vi "Timing.vi"(5 "Tag Values":string[](array[string]), 7 "Tags":string[](array[string]), 8 "error in (no error)":errorcluster, 9 "Time (ms)":u32, 10 "Metric Name":string, 11 "StatD Interface in":refnum<class "StatD Interface.lvclass">) -> (0 "error out":errorcluster, 3 "StatD Interface out":refnum<class "StatD Interface.lvclass">)   [LabVIEW 2011, in "StatD Interface.lvclass"]
doc: "Record a time measurement."
uses:
  StatD Interface.lvclass
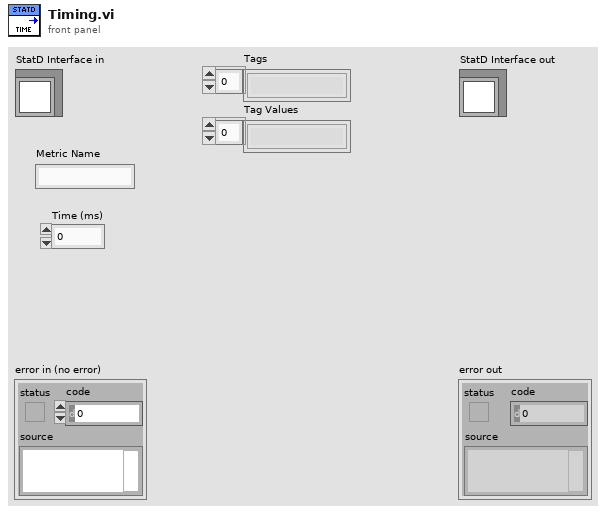
[diagram p1: front panel]
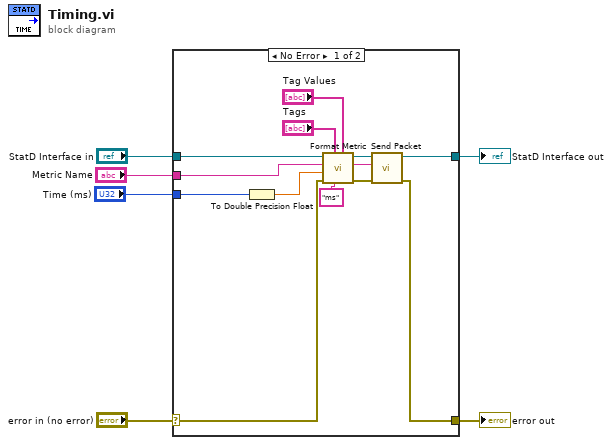
[diagram p0: block diagram]
diagram:
  n1 = case shown="No Error" "error in (no error)" {
    selector: "error in (no error)" -> [w8 w21]
    tunnel: [w18 w21] -> w5
    tunnel: [w19 w20] -> w3
    tunnel: "StatD Interface in" -> [w14 w20]
    tunnel: "Time (ms)" -> [w10 _]
    tunnel: "Metric Name" -> [w9 _]
    frame No Error {
      n2 = To Double Precision Float(number=w10) -> (double precision float=w7:dbl)
      n3 = call "Format Metric.vi"("Tag Values"="Tag Values", "Metric Type"="ms", "Tags"="Tags", "error in (no error)"=w8, "Metric Value"=w7, "Metric Name"=w9, "StatD Interface in"=w14) -> ("error out"=w16:errorcluster, "Packet"=w15:string, "StatD Interface out"=w17:refnum<class "StatD Interface.lvclass">)  [unwired: 2 in]
      n4 = call "Send Packet.vi"("error in (no error)"=w16, "Packet"=w15, "StatD Interface in"=w17) -> ("error out"=w18:errorcluster, "StatD Interface out"=w19:refnum<class "StatD Interface.lvclass">)  [unwired: 7 in]
    }
    frame Error {
    }
  }
  "error out" <- w5
  "StatD Interface out" <- w3
